vi "Channel Set Mapping.vi"(8 "error in (no error)":errorcluster, 10 "Mapping":T2 {"VS Reference" format="%.0x"}, 11 "Item Ref in":T1 format="%.0x") -> (0 "error out":errorcluster, 3 "Item Ref out":T1 format="%.0x")   [LabVIEW 2021, in "Modbus Master System Explorer.lvlib"]
uses:
  Modbus Master System Explorer.lvlib
  <vilib>/NI VeriStand/Custom Device API/Custom Device Item Ref.ctl
  Shared/Controls/Data Model/Mapping.ctl
  Shared/Controls/Data Model/DataType.ctl
  <vilib>/NI VeriStand/Custom Device API/Custom Device API.lvlib
  Shared/Modbus Master Shared.lvlib
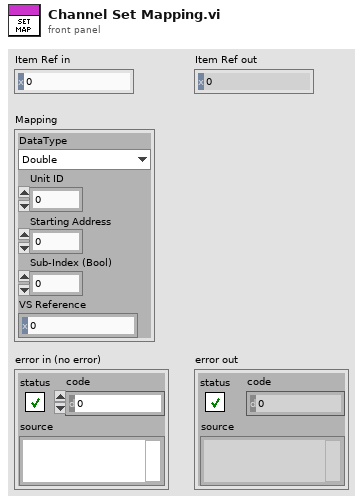
[diagram p1: front panel]
types:
  T1 = typedef "Custom Device API.lvlib/Custom Device Item Ref.ctl" = u64
  T2 = typedef "Modbus Master Shared.lvlib/Mapping.ctl" = cluster{"DataType":T3, "Unit ID":u8, "Starting Address":u16, "Sub-Index (Bool)":u16, "VS Reference":T1}
  T3 = typedef "Modbus Master Shared.lvlib/DataType.ctl" = enum16{"Double", "Single", "I64", "I32", "I16", "I8", "U64", "U32", "U16", "U8", "Boolean"}
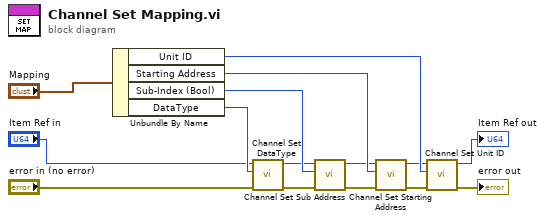
[diagram p0: block diagram]
diagram:
  n1 = Unbundle By Name("Mapping") -> ("Unit ID"=w11:u8, "Starting Address"=w14:u16, "Sub-Index (Bool)"=w13:u16, "DataType"=w12:T3)
  n2 = call "Channel Set DataType.vi"("error in (no error)"="error in (no error)", "DataType"=w12, "Item Ref in"="Item Ref in") -> ("error out"=w9:errorcluster, "Item Ref out"=w10:T1)  [unwired: 7 in]
  n3 = call "Channel Set Sub Address.vi"("error in (no error)"=w9, "Value"=w13, "Item Ref in"=w10) -> ("error out"=w7:errorcluster, "Item Ref out"=w8:T1)  [unwired: 7 in]
  n4 = call "Channel Set Starting Address.vi"("error in (no error)"=w7, "Value"=w14, "Item Ref in"=w8) -> ("error out"=w5:errorcluster, "Item Ref out"=w6:T1)  [unwired: 7 in]
  n5 = call "Channel Set Unit ID.vi"("error in (no error)"=w5, "Value"=w11, "Item Ref in"=w6) -> ("error out"=→"error out":errorcluster, "Item Ref out"=→"Item Ref out":T1)  [unwired: 7 in]
